vi "Test MAIN API.vi"() -> ()   [LabVIEW 2019]
doc: "MAIN API Tester."
uses:
  MICROS.ctl
  MAIN.lvlib
panel:
  in  "MICROS":T1
  in  "VISA resource name":refnum<visa-resource-name>
  in  "Run as Singleton?":bool
  in  "Show Block Diagram":bool
  in  "Refresh Modules":bool
  out "Active Modules":string[](array[string])
  in  "Stop Module":bool
  in  "Select Module":i32(ring)=-1 caption="Select Module\nTo send Request to" items=["All"=-1]
  in  "Run New Module":bool
  in  "Hide Module Panel":bool
  in  "Show Module Panel":bool
  out "Status":string
  # "This VI tests the API for the Module."
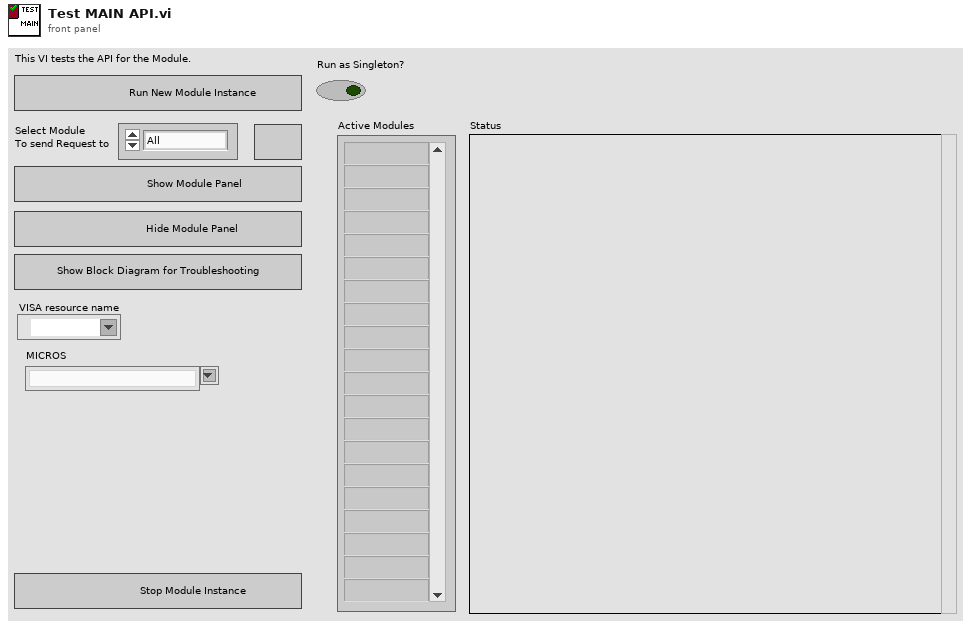
[diagram p1: front panel]
types:
  T1 = typedef "MICROS.ctl" = string
  T2 = typedef "MAIN.lvlib/Broadcast Events--cluster.ctl" = cluster{"Module Did Init":refnum<user-event>, "Status Updated":refnum<user-event>, "Error Reported":refnum<user-event>, "Module Did Stop":refnum<user-event>, "Update Module Execution Status":refnum<user-event>}
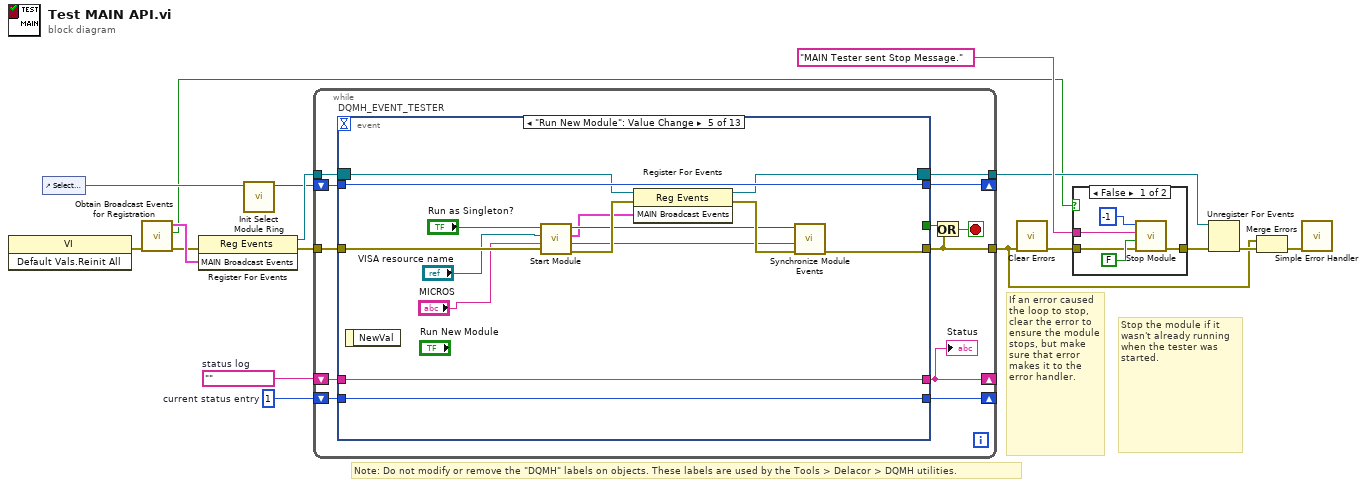
[diagram p0: block diagram]
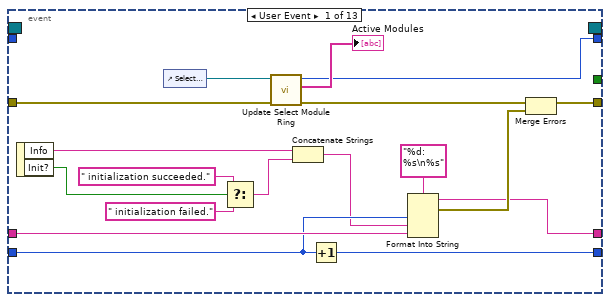
[diagram p3: hidden frame]
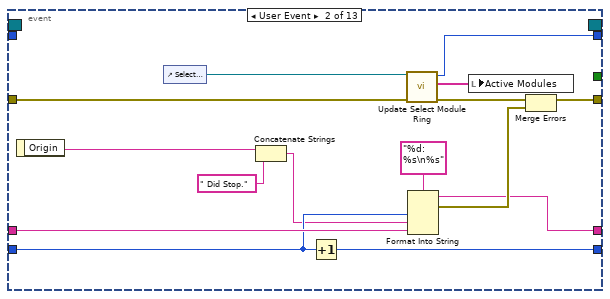
[diagram p4: hidden frame]
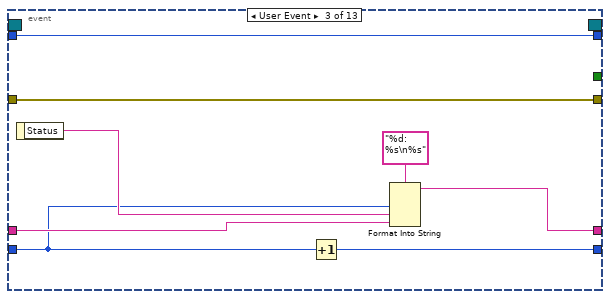
[diagram p5: hidden frame]
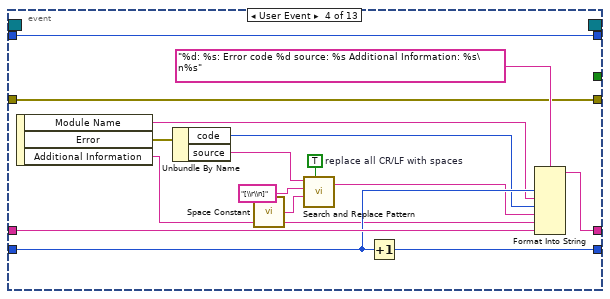
[diagram p6: hidden frame]
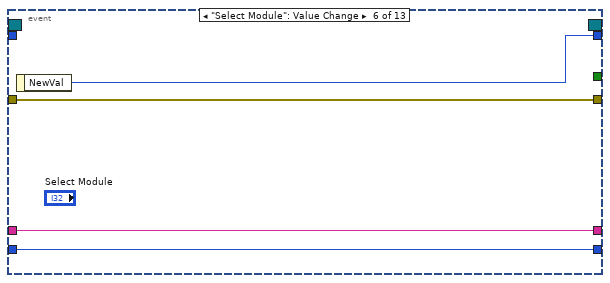
[diagram p7: hidden frame]
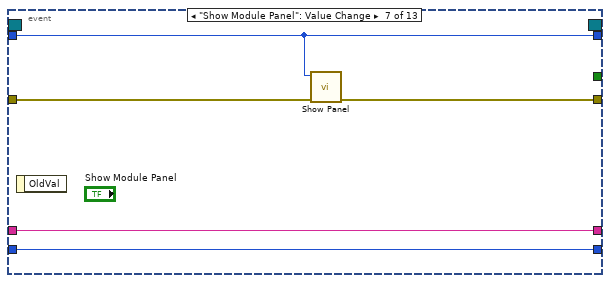
[diagram p8: hidden frame]
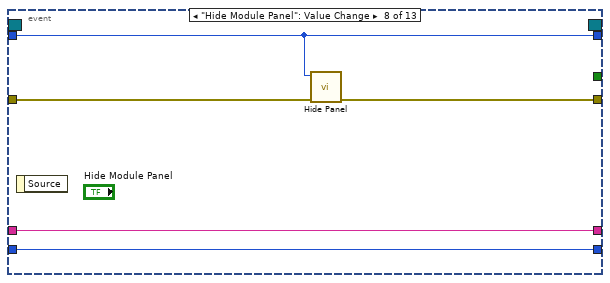
[diagram p9: hidden frame]
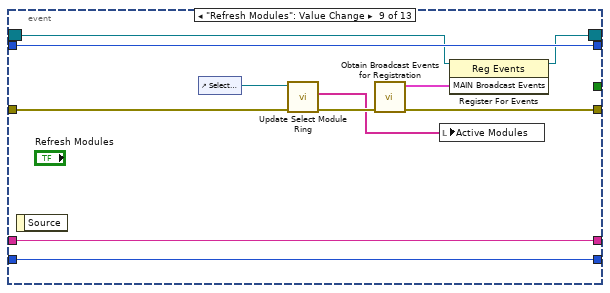
[diagram p10: hidden frame]
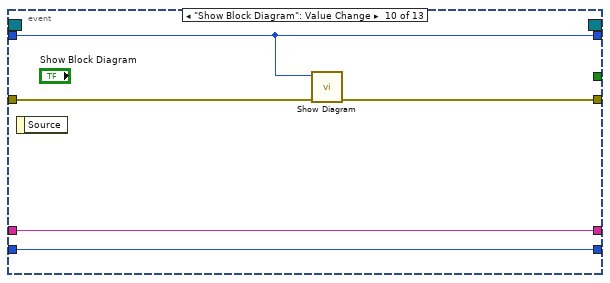
[diagram p11: hidden frame]
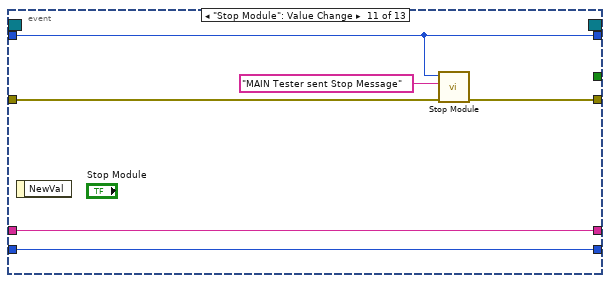
[diagram p12: hidden frame]
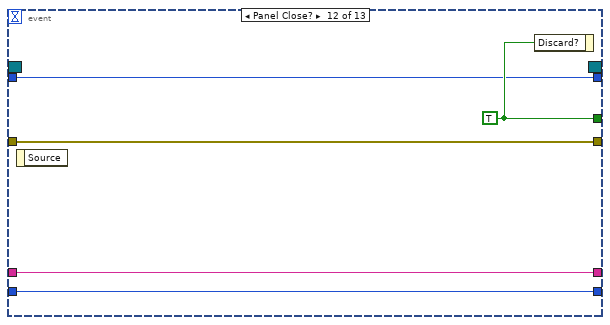
[diagram p13: hidden frame]
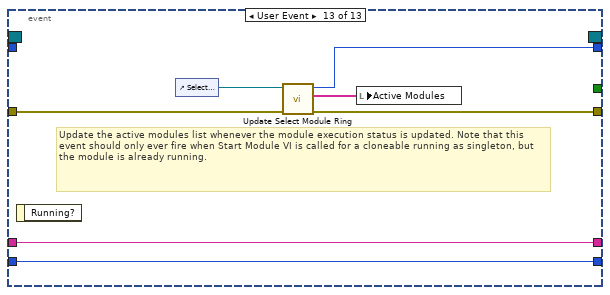
[diagram p14: hidden frame]
diagram:
  w13 = 1  # current status entry
  w14 = ""  # status log
  # "Stop the module if it wasn't already running when the tester was started."
  # "If an error caused the loop to stop, clear the error to ensure the module stops, but make sure that error makes it to the error handler."
  # "Note: Do not modify or remove the \"DQMH\" labels on objects. These labels are used by the Tools > Delacor > DQMH utilities."
  n1 = invoke class="VI" method="Default Vals.Reinit All"() -> (error out=w3:errorcluster)  [unwired: 3 in, 2 out]
  n2 = control-ref of="Select Module"() -> (w11:refnum<vi>)
  n3 = call "Obtain Broadcast Events for Registration.vi"("error in (no error)"=w3) -> ("error out"=w2:errorcluster, "Already running?"=w1:bool, "MAIN Broadcast Events"=w10:T2)  [unwired: 8 in]
  n4 = register-events(error in=w2, w10) -> (reference out=w17:refnum<event-registration>, error out=w9:errorcluster)  [unwired: 1 in]
  n5 = call "Init Select Module Ring.vi"("Select Module Ring Ref"=w11) -> ("Value for All Modules"=w12:i32)  [unwired: 8 in, 2 out]
  n6 = while {
    tunnel: w17 -> [w29]
    tunnel: [w18] -> w4
    tunnel: w9 -> [w27]
    shift-right: [w23] -> _
    shift-left: w14 -> [w25]
    shift-right: [w24] -> _
    shift-left: w13 -> [w26]
    shift-right: [w20] -> _
    shift-left: w12 -> [w21]
    tunnel: [w19] -> w7
    stop <- w22 stop-if-true
    n7 = event "DQMH_EVENT_TESTER" shown="[4] \"Run New Module\": Value Change" {
      selector: w29 -> [_ _ _ _ w95 _ _ _ w121 _ _ _ _]
      dyn-events: [_ _ _ _ w94 _ _ _ w120 _ _ _ _] -> w19
      timeout: _ -> [_ _ _ _ _ _ _ _ _ _ _ _ _]
      tunnel: [_ _ _ _ _ _ _ _ _ _ _ w142 _] -> w28
      tunnel: [w37 w54 w70 w76 w93 w105 w109 w114 w117 w128 w133 w141 w145] -> w18
      tunnel: w27 -> [w39 w56 w70 w76 w96 w105 w110 w115 w122 w131 w134 w141 w146]
      tunnel: w26 -> [w44 w59 w63 w82 w98 w103 w107 w112 w125 w129 w136 w139 w148]
      tunnel: w25 -> [w45 w60 w66 w84 w99 w104 w108 w113 w126 w130 w137 w140 w149]
      tunnel: [w42 w57 w67 w79 w99 w104 w108 w113 w126 w130 w137 w140 w149] -> w23
      tunnel: [w43 w58 w69 w85 w98 w103 w107 w112 w125 w129 w136 w139 w148] -> w24
      tunnel: w21 -> [_ _ w64 w86 w97 _ w106 w111 w124 w127 w135 w138 _]
      tunnel: [w34 w51 w64 w86 w97 w102 w106 w111 w124 w127 w135 w138 w144] -> w20
      event User Event {
        n8 = event-data() -> ("Info"=w41:string, "Init?"=w31:bool)  [unwired: 1 in]
        n9 = control-ref of="Select Module"() -> (w36:refnum<vi>)
        n10 = Select(t=" initialization succeeded.", s=w31, f=" initialization failed.") -> (s? t:f=w30:string)
        n11 = call "Update Select Module Ring.vi"("error in (no error)"=w39, "Select Module Ring Ref"=w36) -> ("error out"=w38:errorcluster, "Active Modules (Array)"=→"Active Modules":string[], "New Module Ring Value"=w34:i32)  [unwired: 7 in]
        n12 = Concatenate Strings(w41, w30) -> (w40:string)
        n13 = Increment(x=w44) -> (x+1=w43:i32)
        n14 = Format Into String(format string="%d: %s\n%s", w44, w40, w45) -> (resulting string=w42:string, error out=w47:errorcluster)  [unwired: 2 in]
        n15 = Merge Errors(w38, w47) -> (w37:errorcluster)
      }
      event User Event {
        n16 = event-data() -> ("Origin"=w49:string)  [unwired: 1 in]
        n17 = control-ref of="Select Module"() -> (w53:refnum<vi>)
        n18 = Concatenate Strings(w49, " Did Stop.") -> (w48:string)
        n19 = Increment(x=w59) -> (x+1=w58:i32)
        n20 = call "Update Select Module Ring.vi"("error in (no error)"=w56, "Select Module Ring Ref"=w53) -> ("error out"=w55:errorcluster, "Active Modules (Array)"=w52:string[], "New Module Ring Value"=w51:i32)  [unwired: 7 in]
        n21 = Format Into String(format string="%d: %s\n%s", w59, w48, w60) -> (resulting string=w57:string, error out=w62:errorcluster)  [unwired: 2 in]
        n22 = local write "Active Modules"(w52) -> ()
        n23 = Merge Errors(w55, w62) -> (w54:errorcluster)
      }
      event User Event {
        n24 = event-data() -> ("Status"=w65:string)  [unwired: 1 in]
        n25 = Increment(x=w63) -> (x+1=w69:i32)
        n26 = Format Into String(format string="%d: %s\n%s", w63, w65, w66) -> (resulting string=w67:string)  [unwired: 2 in, 1 out]
      }
      event User Event {
        w80 = TRUE  # replace all CR/LF with spaces
        n27 = event-data() -> ("Module Name"=w74:string, "Error"=w73:errorcluster, "Additional Information"=w71:string)  [unwired: 1 in]
        n28 = Unbundle By Name(w73) -> ("code"=w75:i32, "source"=w77:string)
        n29 = call <vilib>:"Space Constant.vi"() -> ("String"=w81:string)
        n30 = call <vilib>:"Search and Replace Pattern.vi"("string"=w77, "regular expression (\"\")"="[\\r\\n]" ("regular expression (\"\")"), "replace string (\"\")"=w81, "replace all? (F)"=w80) -> ("result string"=w78:string)  [unwired: 1 in, 1 out]
        n31 = Increment(x=w82) -> (x+1=w85:i32)
        n32 = Format Into String(format string="%d: %s: Error code %d source: %s Additional Information: %s\n%s", w82, w74, w75, w78, w71, w84) -> (resulting string=w79:string)  [unwired: 2 in, 1 out]
      }
      event "Run New Module": Value Change {
        n33 = event-data() -> ()  [unwired: 1 in, 1 out]
        n34 = call "Start Module.vi"("error in (no error)"=w96, "MICROS"="MICROS", "VISA resource name"="VISA resource name", "Run as Singleton? (F)"="Run as Singleton?") -> ("error out"=w100:errorcluster, "Wait for Event Sync?"=w91:bool, "MAIN Broadcast Events"=w90:T2, "Module ID"=w92:i32)  [unwired: 4 in]
        n35 = register-events(reference=w95, error in=w100, w90) -> (reference out=w94:refnum<event-registration>, error out=w101:errorcluster)
        n36 = call "Synchronize Module Events.vi"("error in (no error)"=w101, "Wait for Event Sync?"=w91, "Module ID"=w92) -> ("error out"=w93:errorcluster)  [unwired: 7 in, 1 out]
      }
      event "Select Module": Value Change {
        n37 = event-data() -> ("NewVal"=w102:i32)  [unwired: 1 in]
      }
      event "Show Module Panel": Value Change {
        n38 = event-data() -> ()  [unwired: 1 in, 1 out]
        n39 = call "Show Panel.vi"("error in (no error)"=w110, "Module ID"=w106) -> ("error out"=w109:errorcluster)  [unwired: 9 in]
      }
      event "Hide Module Panel": Value Change {
        n40 = event-data() -> ()  [unwired: 1 in, 1 out]
        n41 = call "Hide Panel.vi"("error in (no error)"=w115, "Module ID"=w111) -> ("error out"=w114:errorcluster)  [unwired: 9 in]
      }
      event "Refresh Modules": Value Change {
        n42 = event-data() -> ()  [unwired: 1 in, 1 out]
        n43 = control-ref of="Select Module"() -> (w123:refnum<vi>)
        n44 = call "Update Select Module Ring.vi"("error in (no error)"=w122, "Select Module Ring Ref"=w123) -> ("error out"=w118:errorcluster, "Active Modules (Array)"=w116:string[])  [unwired: 7 in, 1 out]
        n45 = call "Obtain Broadcast Events for Registration.vi"("error in (no error)"=w118) -> ("error out"=w117:errorcluster, "MAIN Broadcast Events"=w119:T2)  [unwired: 8 in, 1 out]
        n46 = local write "Active Modules"(w116) -> ()
        n47 = register-events(reference=w121, w119) -> (reference out=w120:refnum<event-registration>)  [unwired: 1 in, 1 out]
      }
      event "Show Block Diagram": Value Change {
        n48 = event-data() -> ()  [unwired: 1 in, 1 out]
        n49 = call "Show Diagram.vi"("error in (no error)"=w131, "Module ID"=w127) -> ("error out"=w128:errorcluster)  [unwired: 9 in]
      }
      event "Stop Module": Value Change {
        n50 = event-data() -> ()  [unwired: 1 in, 1 out]
        n51 = call "Stop Module.vi"("error in (no error)"=w134, "Origin"="MAIN Tester sent Stop Message", "Module ID"=w135) -> ("error out"=w133:errorcluster)  [unwired: 8 in]
      }
      event Panel Close? {
        w142 = TRUE ("Discard?")
        n52 = event-data() -> ()  [unwired: 1 in, 1 out]
        n53 = event-data("Discard?"=w142) -> ()  [unwired: 1 in, 1 out]
      }
      event User Event {
        # "Update the active modules list whenever the module execution status is updated. Note that this event should only ever fire when Start Module VI is called for a cloneable running as singleton, but the module is already running."
        n54 = event-data() -> ()  [unwired: 1 in, 1 out]
        n55 = control-ref of="Select Module"() -> (w147:refnum<vi>)
        n56 = call "Update Select Module Ring.vi"("error in (no error)"=w146, "Select Module Ring Ref"=w147) -> ("error out"=w145:errorcluster, "Active Modules (Array)"=w143:string[], "New Module Ring Value"=w144:i32)  [unwired: 7 in]
        n57 = local write "Active Modules"(w143) -> ()
      }
    }
    "Status" <- w23
    n58 = Or(x=w28, y=w18) -> (x .or. y?=w22:bool)
  }
  n59 = call <vilib>:"Clear Errors.vi"("error in (no error)"=w4) -> ("error out"=w6:errorcluster)  [unwired: 5 in, 1 out]
  n60 = case shown="False" w1 {
    tunnel: [w154 w155] -> w15
    tunnel: "MAIN Tester sent Stop Message." ("Origin") -> [w153 _]
    tunnel: w6 -> [w150 w155]
    frame False {
      n61 = call "Stop Module.vi"("error in (no error)"=w150, "Wait for Module to stop? (F)"=FALSE ("Wait for Module to stop?"), "Origin"=w153, "Module ID"=-1 ("Stop all")) -> ("error out"=w154:errorcluster)  [unwired: 7 in]
    }
    frame True {
    }
  }
  n62 = Unregister For Events(event registration refnum=w7, error in=w15) -> (error out=w16:errorcluster)
  n63 = Merge Errors(w4, w16) -> (w5:errorcluster)
  n64 = call <vilib>:"Simple Error Handler.vi"("error in (no error)"=w5) -> ()  [unwired: 4 in, 5 out]
